vi "verticalmenuRecovery.vi"() -> ()   [LabVIEW 2011]
uses:
  GlobalPath.vi
  MyData/MicroMegas/ProgrammiMDT/DefGlobal/GlobalData.vi
  GlobalVi.vi
panel:
  in  "CheckPress":bool
  in  "CheckAmbient":bool
  in  "StartPress":bool
  out "file path":path=path "g:/user/assembly/Restart.txt"
  in  "StartPanel":bool
  in  "CheckLogFile":bool
  out "last program\nbackup":string
  out "Check":path=path "g:/user/assembly/checkcrash.txt"
  in  "stop":bool
  in  "StartAmbient":bool
  # "MM Pavia"
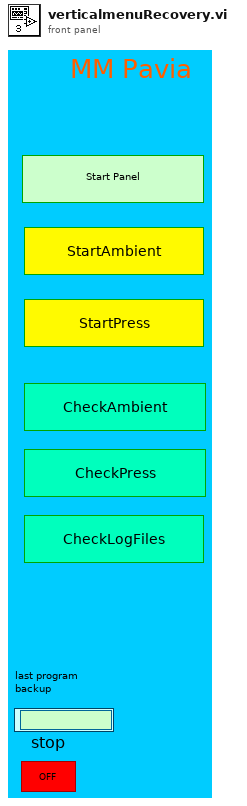
[diagram p1: front panel]
types:
  T1 = enum16{"open", "open or create", "create or replace", "create"}
  T2 = cluster{"top":i32, "left":i32, "bottom":i32, "right":i32}
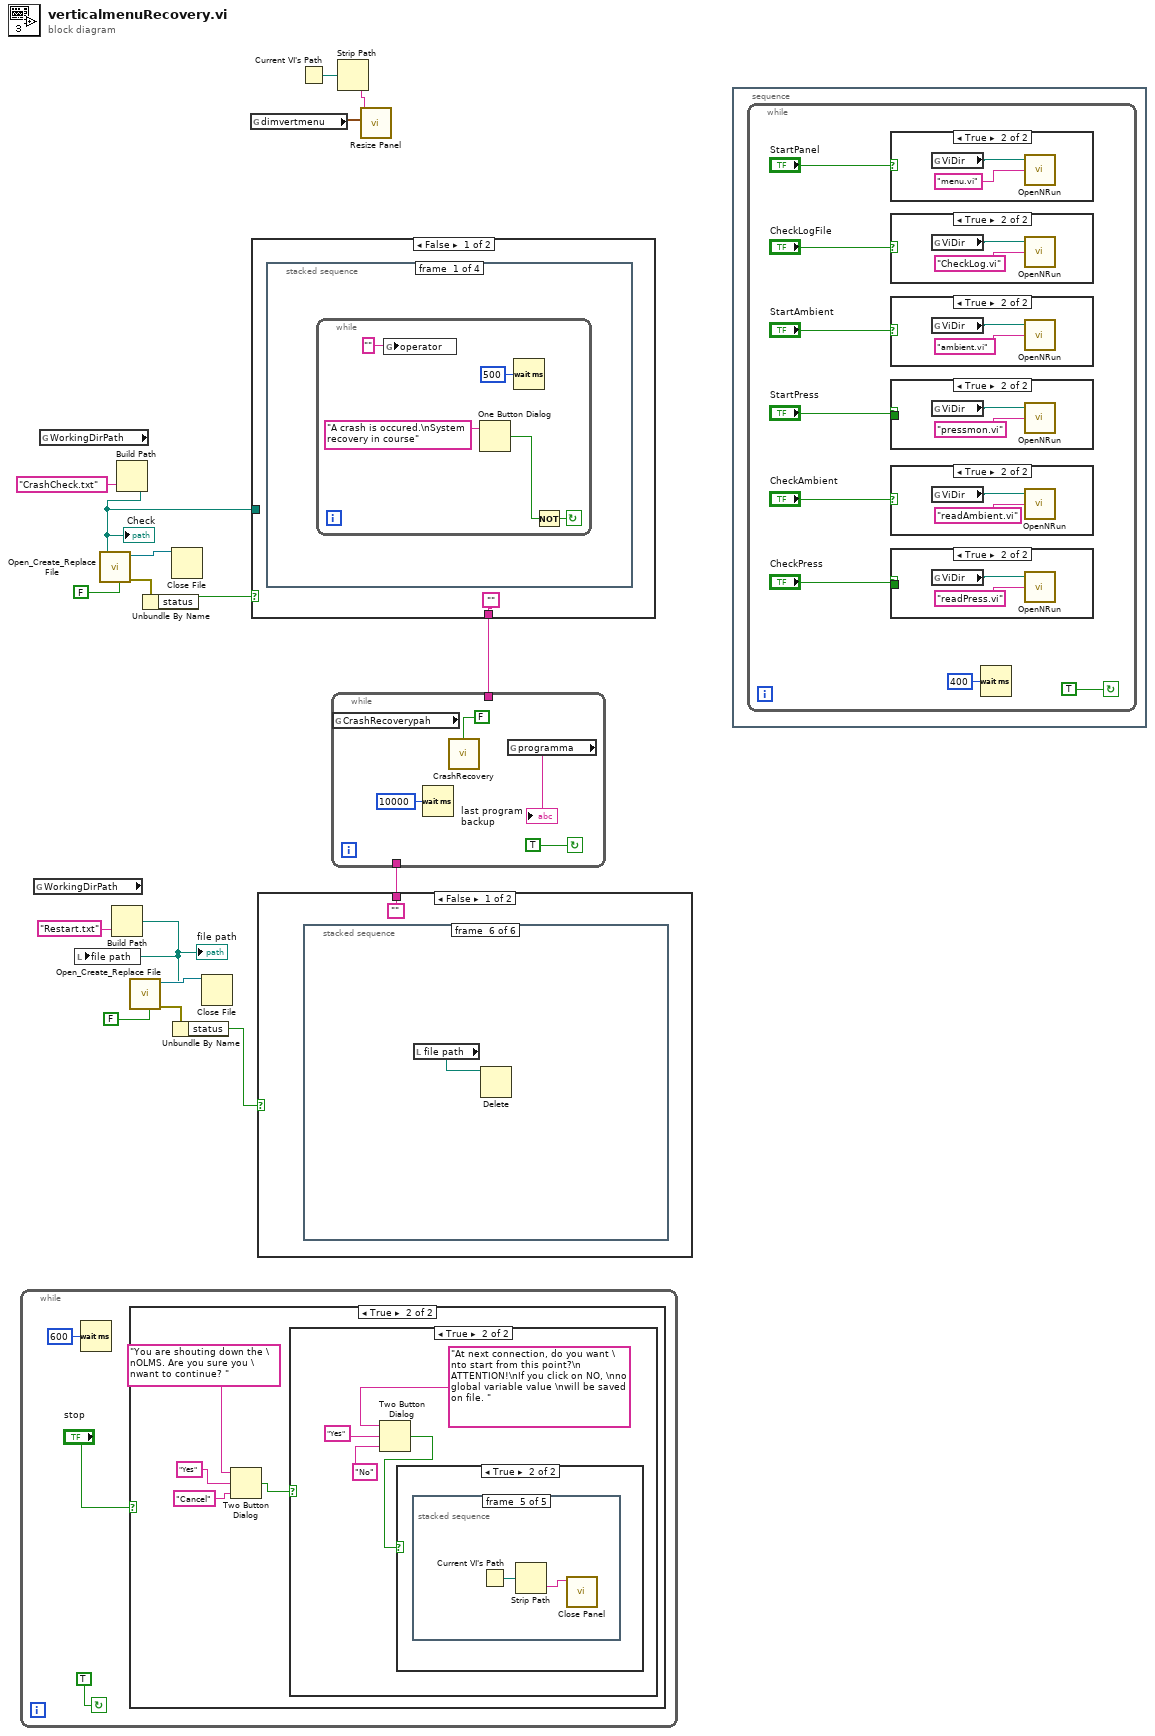
[diagram p0: block diagram]
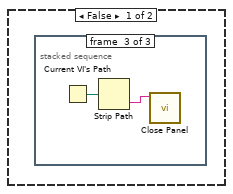
[diagram p4: hidden frame]
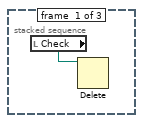
[diagram p5: hidden frame]
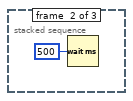
[diagram p6: hidden frame]
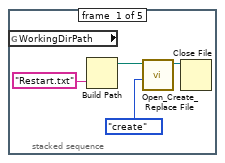
[diagram p7: hidden frame]
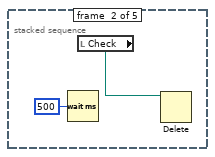
[diagram p8: hidden frame]
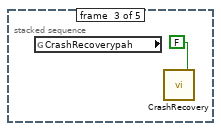
[diagram p9: hidden frame]
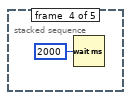
[diagram p10: hidden frame]
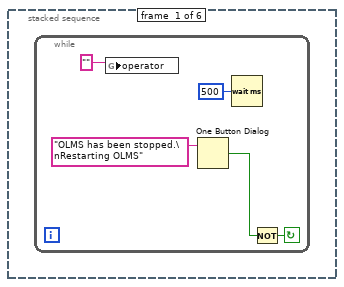
[diagram p17: hidden frame]
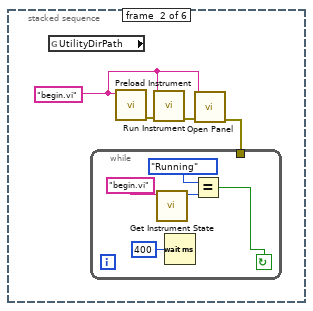
[diagram p18: hidden frame]
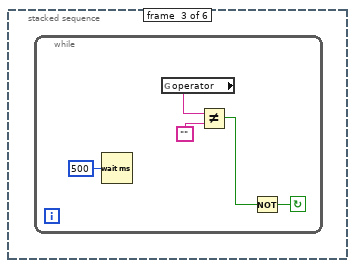
[diagram p19: hidden frame]
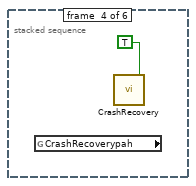
[diagram p20: hidden frame]
diagram:
  n1 = while {
    stop <- TRUE continue-if-true
    n2 = Wait (ms)(milliseconds to wait=u32 600) -> ()  [unwired: 1 out]
    n3 = case shown="True" "stop" {
      frame False {
      }
      frame True {
        n4 = Two Button Dialog(message="You are shouting down the \nOLMS. Are you sure you \nwant to continue? ", 1:"Cancel" ("F button name (\"Cancel\")"), 2:"Yes" ("T button name (\"OK\")")) -> (T button?=w21:bool)
        n5 = case shown="True" w21 {
          frame False {
          }
          frame True {
            n6 = Two Button Dialog(message="At next connection, do you want \nto start from this point?\n ATTENTION!\nIf you click on NO, \nno global variable value \nwill be saved on file. ", 1:"No" ("F button name (\"Cancel\")"), 2:"Yes" ("T button name (\"OK\")")) -> (T button?=w25:bool)
            n7 = case shown="True" w25 {
              frame False {
                n8 = stacked-sequence {
                  frame #0 {
                    n9 = local read "Check"() -> (w29:path)
                    n10 = Delete(path (use dialog)=w29) -> ()  [unwired: 4 in, 3 out]
                  }
                  frame #1 {
                    n11 = Wait (ms)(milliseconds to wait=u32 500) -> ()  [unwired: 1 out]
                  }
                  frame #2 {
                    n12 = Current VI's Path() -> (path=w32:path)
                    n13 = Strip Path(path=w32) -> (name=w31:string)  [unwired: 1 out]
                    n14 = call <vilib>:"Close Panel.vi"("VI name"=w31) -> ()  [unwired: 10 in, 1 out]
                  }
                }
              }
              frame True {
                n15 = stacked-sequence {
                  frame #0 {
                    n16 = global read "GlobalPath.vi" "WorkingDirPath"() -> ()  [unwired: 1 out]
                    n17 = Build Path(name or relative path="Restart.txt") -> (appended path=w33:path)  [unwired: 1 in]
                    n18 = call <vilib>:"Open_Create_Replace File.vi"("function (open:0)"=T1."create", "file path"=w33) -> ("refnum"=w35:refnum<file>)  [unwired: 6 in, 3 out]
                    n19 = Close File(refnum=w35) -> ()  [unwired: 1 in, 2 out]
                  }
                  frame #1 {
                    n20 = Wait (ms)(milliseconds to wait=u32 500) -> ()  [unwired: 1 out]
                    n21 = local read "Check"() -> (w38:path)
                    n22 = Delete(path (use dialog)=w38) -> ()  [unwired: 4 in, 3 out]
                  }
                  frame #2 {
                    n23 = global read "GlobalPath.vi" "CrashRecoverypah"() -> ()  [unwired: 1 out]
                    n24 = call "CrashRecovery.vi"("Boolean"=FALSE) -> ()  [unwired: 1 in]
                  }
                  frame #3 {
                    n25 = Wait (ms)(milliseconds to wait=u32 2000) -> ()  [unwired: 1 out]
                  }
                  frame #4 {
                    n26 = Current VI's Path() -> (path=w41:path)
                    n27 = Strip Path(path=w41) -> (name=w42:string)  [unwired: 1 out]
                    n28 = call <vilib>:"Close Panel.vi"("VI name"=w42) -> ()  [unwired: 10 in, 1 out]
                  }
                }
              }
            }
          }
        }
      }
    }
  }
  n29 = global read "GlobalPath.vi" "WorkingDirPath"() -> ()  [unwired: 1 out]
  n30 = global read "GlobalPath.vi" "WorkingDirPath"() -> ()  [unwired: 1 out]
  n31 = Build Path(name or relative path="Restart.txt") -> (appended path=w1:path)  [unwired: 1 in]
  "file path" <- w1
  n32 = local write "file path"(w1) -> ()
  n33 = Build Path(name or relative path="CrashCheck.txt") -> (appended path=w3:path)  [unwired: 1 in]
  "Check" <- w3
  n34 = call <vilib>:"Open_Create_Replace File.vi"("advisory dialog? (display:T)"=FALSE, "file path"=w3) -> ("error out"=w15:errorcluster, "refnum"=w12:refnum<file>)  [unwired: 6 in, 2 out]
  n35 = call <vilib>:"Open_Create_Replace File.vi"("advisory dialog? (display:T)"=FALSE, "file path"=w1) -> ("error out"=w10:errorcluster, "refnum"=w8:refnum<file>)  [unwired: 6 in, 2 out]
  n36 = Unbundle By Name(w15) -> ("status"=w14:bool)
  n37 = Close File(refnum=w12) -> ()  [unwired: 1 in, 2 out]
  n38 = Unbundle By Name(w10) -> ("status"=w7:bool)
  n39 = Close File(refnum=w8) -> ()  [unwired: 1 in, 2 out]
  n40 = global read "GlobalVi.vi" "dimvertmenu"() -> (w5:T2)
  n41 = case shown="False" w14 {
    tunnel: w3 -> [_ w69]
    tunnel: ["" ""] -> w11
    frame False {
      n42 = stacked-sequence {
        frame #0 {
          n43 = while {
            stop <- w45 continue-if-true
            n44 = global write "GlobalData.vi" "operator"("" ("operator")) -> ()
            n45 = One Button Dialog(message="A crash is occured.\nSystem recovery in course") -> (true=w46:bool)  [unwired: 1 in]
            n46 = Wait (ms)(milliseconds to wait=u32 500) -> ()  [unwired: 1 out]
            n47 = Not(x=w46) -> (.not. x?=w45:bool)
          }
        }
        frame #1 {
          w52 = "begin.vi"
          n48 = global read "GlobalPath.vi" "UtilityDirPath"() -> ()  [unwired: 1 out]
          n49 = call <vilib>:"Preload Instrument.vi"("VI name"=w52) -> ("error out"=w51:errorcluster)  [unwired: 10 in]
          n50 = call <vilib>:"Run Instrument.vi"("error in (no error)"=w51, "VI name"=w52) -> ("error out"=w50:errorcluster)  [unwired: 9 in]
          n51 = call <vilib>:"Open Panel.vi"("error in (no error)"=w50, "VI name"=w52) -> ("error out"=w49:errorcluster)  [unwired: 9 in]
          n52 = while {
            tunnel: w49 -> [_]
            stop <- w53 continue-if-true
            n53 = call <vilib>:"Get Instrument State.vi"("VI name"="begin.vi") -> ("vi state"=w55:enum32{"Broken", "Idle", "Running"})  [unwired: 8 in, 2 out]
            n54 = Wait (ms)(milliseconds to wait=u32 400 ("millisecond multiple")) -> ()  [unwired: 1 out]
            n55 = Equal?(x=enum32{"Broken", "Idle", "Running"}."Running", y=w55) -> (x = y?=w53:bool)
          }
        }
        frame #2 {
          n56 = while {
            stop <- w61 continue-if-true
            n57 = global read "GlobalData.vi" "operator"() -> (w58:string)
            n58 = Wait (ms)(milliseconds to wait=u32 500) -> ()  [unwired: 1 out]
            n59 = Not Equal?(x=w58, y="") -> (x != y?=w59:bool)
            n60 = case shown="True" w59 {
              tunnel: w59 -> [_ w63]
              frame False {
              }
              frame True {
                n61 = global read "GlobalPath.vi" "CrashRecoverypah"() -> ()  [unwired: 1 out]
                n62 = call "CrashRecovery.vi"("Boolean"=w63) -> ()  [unwired: 1 in]
              }
            }
            n63 = Not(x=w59) -> (.not. x?=w61:bool)
          }
        }
        frame #3 {
          n64 = global read "GlobalData.vi" "CurrentDir"() -> (w64:path)
          n65 = global read "GlobalData.vi" "programma"() -> (w65:string)
          n66 = call <vilib>:"Preload Instrument.vi"("VI path"=w64, "VI name"=w65) -> ("error out"=w67:errorcluster)  [unwired: 9 in]
          n67 = call <vilib>:"Run Instrument.vi"("error in (no error)"=w67, "VI name"=w65) -> ("error out"=w66:errorcluster)  [unwired: 9 in]
          n68 = call <vilib>:"Open Panel.vi"("error in (no error)"=w66, "VI name"=w65) -> ()  [unwired: 9 in, 1 out]
        }
      }
    }
    frame True {
      n69 = call <vilib>:"Open_Create_Replace File.vi"("function (open:0)"=T1."create", "file path"=w69) -> ("refnum"=w70:refnum<file>)  [unwired: 6 in, 3 out]
      n70 = Close File(refnum=w70) -> ()  [unwired: 1 in, 2 out]
    }
  }
  n71 = case shown="False" w7 {
    tunnel: ["" ""] -> w6
    frame False {
      n72 = stacked-sequence {
        frame #0 {
          n73 = while {
            stop <- w75 continue-if-true
            n74 = global write "GlobalData.vi" "operator"("" ("operator")) -> ()
            n75 = One Button Dialog(message="OLMS has been stopped.\nRestarting OLMS") -> (true=w76:bool)  [unwired: 1 in]
            n76 = Wait (ms)(milliseconds to wait=u32 500) -> ()  [unwired: 1 out]
            n77 = Not(x=w76) -> (.not. x?=w75:bool)
          }
        }
        frame #1 {
          w81 = "begin.vi"
          n78 = global read "GlobalPath.vi" "UtilityDirPath"() -> ()  [unwired: 1 out]
          n79 = call <vilib>:"Preload Instrument.vi"("VI name"=w81) -> ("error out"=w80:errorcluster)  [unwired: 10 in]
          n80 = call <vilib>:"Run Instrument.vi"("error in (no error)"=w80, "VI name"=w81) -> ("error out"=w79:errorcluster)  [unwired: 9 in]
          n81 = call <vilib>:"Open Panel.vi"("error in (no error)"=w79, "VI name"=w81) -> ("error out"=w78:errorcluster)  [unwired: 9 in]
          n82 = while {
            tunnel: w78 -> [_]
            stop <- w82 continue-if-true
            n83 = call <vilib>:"Get Instrument State.vi"("VI name"="begin.vi") -> ("vi state"=w84:enum32{"Broken", "Idle", "Running"})  [unwired: 8 in, 2 out]
            n84 = Wait (ms)(milliseconds to wait=u32 400 ("millisecond multiple")) -> ()  [unwired: 1 out]
            n85 = Equal?(x=enum32{"Broken", "Idle", "Running"}."Running", y=w84) -> (x = y?=w82:bool)
          }
        }
        frame #2 {
          n86 = while {
            stop <- w90 continue-if-true
            n87 = Wait (ms)(milliseconds to wait=u32 500) -> ()  [unwired: 1 out]
            n88 = global read "GlobalData.vi" "operator"() -> (w87:string)
            n89 = Not Equal?(x=w87, y="") -> (x != y?=w88:bool)
            n90 = Not(x=w88) -> (.not. x?=w90:bool)
          }
        }
        frame #3 {
          n91 = global read "GlobalPath.vi" "CrashRecoverypah"() -> ()  [unwired: 1 out]
          n92 = call "CrashRecovery.vi"("Boolean"=TRUE) -> ()  [unwired: 1 in]
        }
        frame #4 {
          n93 = global read "GlobalData.vi" "CurrentDir"() -> (w93:path)
          n94 = global read "GlobalData.vi" "programma"() -> (w94:string)
          n95 = call <vilib>:"Preload Instrument.vi"("VI path"=w93, "VI name"=w94) -> ("error out"=w96:errorcluster)  [unwired: 9 in]
          n96 = call <vilib>:"Run Instrument.vi"("error in (no error)"=w96, "VI name"=w94) -> ("error out"=w95:errorcluster)  [unwired: 9 in]
          n97 = call <vilib>:"Open Panel.vi"("error in (no error)"=w95, "VI name"=w94) -> ()  [unwired: 9 in, 1 out]
        }
        frame #5 {
          n98 = local read "file path"() -> (w97:path)
          n99 = Delete(path (use dialog)=w97) -> ()  [unwired: 4 in, 3 out]
        }
      }
    }
    frame True {
    }
  }
  n100 = Current VI's Path() -> (path=w17:path)
  n101 = while {
    tunnel: w6 -> [_]
    tunnel: w11 -> [_]
    stop <- TRUE continue-if-true
    n102 = global read "GlobalPath.vi" "CrashRecoverypah"() -> ()  [unwired: 1 out]
    n103 = Wait (ms)(milliseconds to wait=u32 10000) -> ()  [unwired: 1 out]
    n104 = call "CrashRecovery.vi"("Boolean"=FALSE) -> ()  [unwired: 1 in]
    n105 = global read "GlobalData.vi" "programma"() -> (→"last program\nbackup":string)
  }
  n106 = Strip Path(path=w17) -> (name=w16:string)  [unwired: 1 out]
  n107 = call <vilib>:"Resize Panel.vi"("panel location and size"=w5, "VI name"=w16) -> ()  [unwired: 9 in, 1 out]
  n108 = stacked-sequence {
    frame #0 {
      n109 = while {
        stop <- TRUE continue-if-true
        n110 = case shown="True" "StartPanel" {
          frame False {
          }
          frame True {
            n111 = global read "GlobalPath.vi" "ViDir"() -> (w122:path)
            n112 = call "OpenNRun.vi"("VI name"="menu.vi", "ViDirPath"=w122) -> ()  [unwired: 1 in]
          }
        }
        n113 = case shown="True" "CheckLogFile" {
          frame False {
          }
          frame True {
            n114 = global read "GlobalPath.vi" "ViDir"() -> (w120:path)
            n115 = call "OpenNRun.vi"("VI name"="CheckLog.vi", "ViDirPath"=w120) -> ()  [unwired: 1 in]
          }
        }
        n116 = case shown="True" "StartAmbient" {
          frame False {
          }
          frame True {
            n117 = global read "GlobalPath.vi" "ViDir"() -> (w118:path)
            n118 = call "OpenNRun.vi"("VI name"="ambient.vi", "ViDirPath"=w118) -> ()  [unwired: 1 in]
          }
        }
        n119 = case shown="True" {
          selector: _ -> [_ _]
          tunnel: "StartPress" -> [_ _]
          frame False {
          }
          frame True {
            n120 = global read "GlobalPath.vi" "ViDir"() -> (w116:path)
            n121 = call "OpenNRun.vi"("VI name"="pressmon.vi", "ViDirPath"=w116) -> ()  [unwired: 1 in]
          }
        }
        n122 = case shown="True" "CheckAmbient" {
          frame False {
          }
          frame True {
            n123 = global read "GlobalPath.vi" "ViDir"() -> (w114:path)
            n124 = call "OpenNRun.vi"("VI name"="readAmbient.vi", "ViDirPath"=w114) -> ()  [unwired: 1 in]
          }
        }
        n125 = case shown="True" {
          selector: _ -> [_ _]
          tunnel: "CheckPress" -> [_ _]
          frame False {
          }
          frame True {
            n126 = global read "GlobalPath.vi" "ViDir"() -> (w112:path)
            n127 = call "OpenNRun.vi"("VI name"="readPress.vi", "ViDirPath"=w112) -> ()  [unwired: 1 in]
          }
        }
        n128 = Wait (ms)(milliseconds to wait=u32 400 ("millisecond multiple")) -> ()  [unwired: 1 out]
      }
    }
  }
